vi "CMN_Arr2Str.vi"(10 "Array in":string[](array[string])) -> (2 "string out":string)   [LabVIEW 2016]
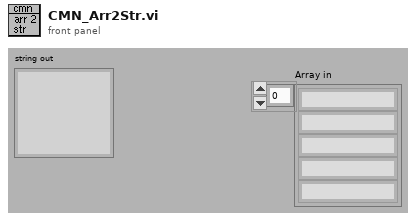
[diagram p1: front panel]
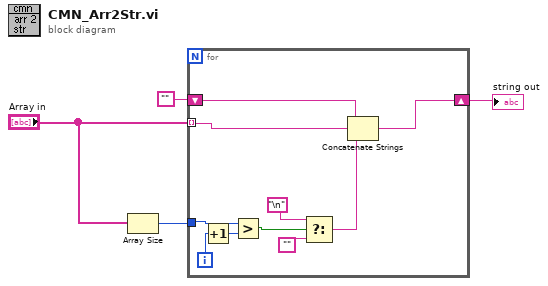
[diagram p0: block diagram]
diagram:
  n1 = Array Size(array="Array in") -> (size(s)=w1:i32)
  n2 = for {
    tunnel: "Array in" -> [w12] mode=indexing
    shift-right: [w14] -> w3
    shift-left: "" -> [w13]
    tunnel: w1 -> [w11]
    i -> [w10]
    n3 = Increment(x=w10) -> (x+1=w6:i32)
    n4 = Greater?(x=w11, y=w6) -> (0:w9:bool)
    n5 = Select(t="\n", s=w9, f="") -> (s? t:f=w7:string)
    n6 = Concatenate Strings(w13, w12, w7) -> (w14:string)
  }
  "string out" <- w3
